vi "Read Required Keys.vi"(8 "error in (no error)":errorcluster, 11 "Instruments in":refnum<class "Instruments.lvclass">) -> (0 "error out":errorcluster, 2 "Required Keys":string[](array[string]), 3 "Instruments out":refnum<class "Instruments.lvclass">)   [LabVIEW 2023, in "Instruments.lvlib" / "Instruments.lvclass"]
doc: "<b>Instruments </b>\nAt this layer additional information is necessary to define instrument functionality universally\n\n<b>Keys</b>\n<b>Calibration</b> - Calibration Due Date (NCR = No Cal Required)\n<b>Resource</b> - String representation of the connection resource \n<b>Poll(ms)</b> - Measurement Query interval (how often should the GUI update with telemetry)\n<b>Panel</b> - Docking Position of the instrument in the manual GUI\n<b>Simulated</b> - True/False is this implementation an simulated instrument?\n<b>Enabled</b> - Enabled - This allows developers to integrate the test instruments in stages"
uses:
  Library/Instruments.lvclass
  Custom Controls/Configuration Keys.ctl
  builds/Framework/Configuration.lvlibp/Library/Configuration.lvclass
  Library/Instruments.lvclass/Instruments.ctl
panel:
  in  "Configuration Keys":T1
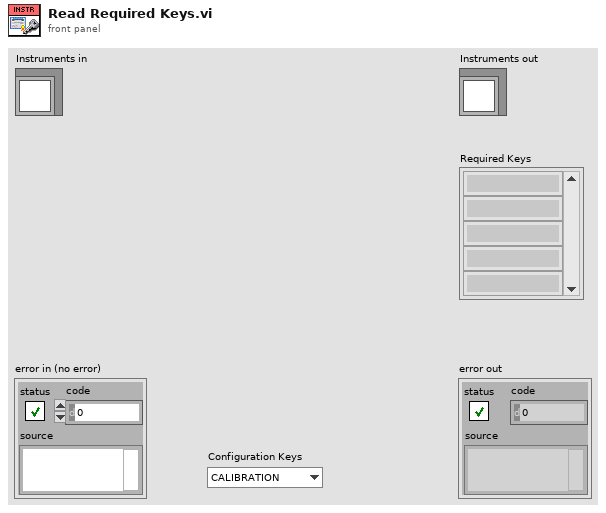
[diagram p1: front panel]
types:
  T1 = typedef "Instruments.lvlib/Instruments.lvclass/Configuration Keys.ctl" = enum16{"CALIBRATION", "RESOURCE", "POLL(MS)", "PANEL", "SIMULATED", "ENABLED"}
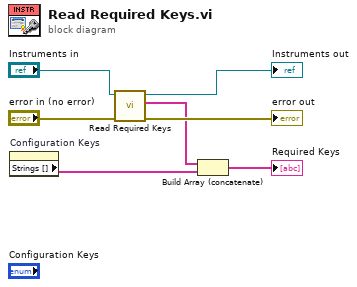
[diagram p0: block diagram]
diagram:
  n1 = property on="Configuration Keys" class="Enum (strict)"() -> ("Strings []"=w2:string[])  [unwired: 2 in, 2 out]
  n2 = call-parent "Read Required Keys.vi"("error in (no error)"="error in (no error)", "Configuration in"="Instruments in") -> ("error out"=→"error out":errorcluster, "Required Keys"=w3:string[], "Configuration out"=→"Instruments out":refnum<class "Instruments.lvclass">)  [unwired: 7 in]
  n3 = Build Array (concatenate)(w3, w2) -> (→"Required Keys":string[])
